vi "Initialize Front Panel.vi"(8 "error in (no error)":errorcluster, 11 "Subroutine Loop Dialog in":refnum<class "Subroutine Dialog.lvclass">) -> (0 "error out":errorcluster, 3 "For Loop Dialog out":refnum<class "Subroutine Dialog.lvclass">)   [LabVIEW 2019, in "Subroutine Dialog.lvclass"]
doc: "<License>\nCopyright © 2017 Composed Systems, LLC | All rights reserved\nwww.composed.io\n\nAuthor: Ethan Stern <ethan.stern@composed.io>\n\nThis software is provided \"AS IS\" WITHOUT WARRANTIES, either express or implied, AND IS FOR EDUCATIONAL PURPOSES ONLY.\n</License>"
uses:
  <vilib>/gpm_packages/@cs/Test-executive-builder/Source/Test Executive Builder Dialogs/Edit Subroutine Dialog/Subroutine Dialog.lvclass
  C:/Program Files/National Instruments/LabVIEW 2019/vi.lib/gpm_packages/@cs/popup-viewmanager/Source/Popup ViewManager/Popup ViewManager.lvclass
  <vilib>/gpm_packages/@cs/Test-executive-builder/Source/Test Executive Builder Dialogs/Edit Subroutine Dialog/Subroutine Dialog.lvclass/Subroutine Dialog.ctl
  <vilib>/gpm_packages/@cs/mva-viewable/Source/IViewable/IViewable Messages/Insert Front Panel Msg/Insert Front Panel Msg.lvclass/Insert Front Panel Msg.ctl
  <vilib>/ActorFramework/Message Enqueuer/Message Enqueuer.lvclass/Message Enqueuer.ctl
  <vilib>/gpm_packages/@cs/Test-executive-builder/Source/Test Executive Builder Dialogs/IAttribute Data Type View Messages/Set Value Msg/Set Value Msg.lvclass/Set Value Msg.ctl
  <vilib>/ActorFramework/Message Enqueuer/Enqueue.vi
  <vilib>/gpm_packages/@cs/mva-viewable/Source/IViewable/IViewable Messages/Insert Front Panel Msg/Insert Front Panel Msg.lvclass
  C:/Program Files/National Instruments/LabVIEW 2019/vi.lib/ActorFramework/Message/Message.lvclass
  <vilib>/gpm_packages/@cs/Test-executive-builder/Source/Test Executive Builder Dialogs/IAttribute Data Type View Messages/Set Value Msg/Set Value Msg.lvclass
  <vilib>/ActorFramework/Message Priority Queue/Priority Enqueue.vi
  <vilib>/gpm_packages/@cs/Test-executive-builder/Source/Test Executive Builder Dialogs/ITest Executive Builder Dialog/ITest Executive Builder Dialog.lvclass
  <vilib>/gpm_packages/@cs/popup-viewmanager/Source/Popup ViewManager/Popup ViewManager.lvclass
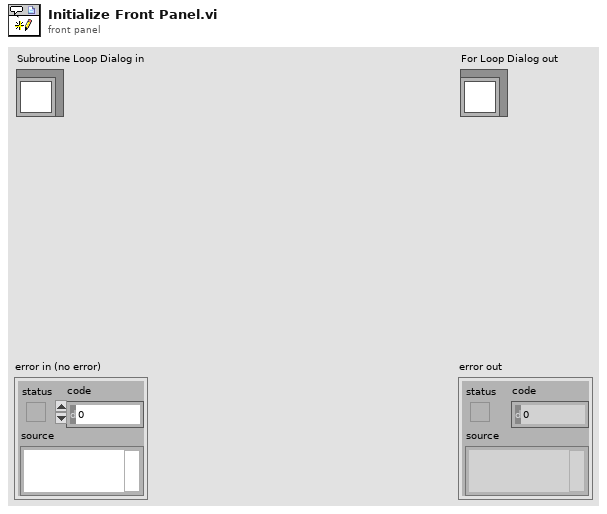
[diagram p1: front panel]
types:
  T1 = typedef "IViewable.lvlib/ProtectedSubpanel.lvclass/Protected Subpanel Reference.ctl" = refnum<data-value>
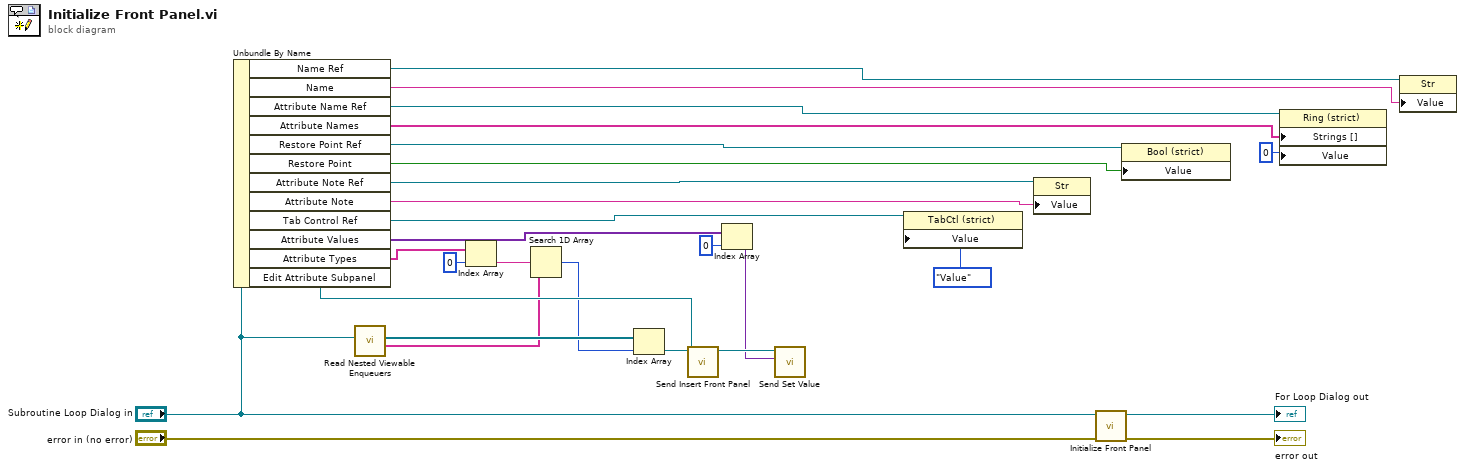
[diagram p0: block diagram]
diagram:
  n1 = Unbundle By Name("Subroutine Loop Dialog in") -> ("Name Ref"=w25:refnum<vi>, "Name"=w24:string, "Attribute Name Ref"=w22:refnum<vi>, "Attribute Names"=w21:string[], "Restore Point Ref"=w19:refnum<vi>, "Restore Point"=w18:bool, "Attribute Note Ref"=w17:refnum<vi>, "Attribute Note"=w16:string, "Tab Control Ref"=w11:refnum<vi>, "Attribute Values"=w2:variant[], "Attribute Types"=w9:string[], "Edit Attribute Subpanel"=w12:T1)
  n2 = call <vilib>:"Read Nested Viewable Enqueuers.vi"("Popup ViewManager in"="Subroutine Loop Dialog in") -> ("Viewable Names"=w7:string[], "Nested Enqueuers"=w14:refnum<class "Message Enqueuer.lvclass">[])  [unwired: 9 in]
  n3 = Index Array(array=w9, index=0) -> (element=w6:string)
  n4 = Search 1D Array(1D array=w7, element=w6) -> (index of element=w5:i32)  [unwired: 1 in]
  n5 = Index Array(array=w14, index=w5) -> (element=w13:refnum<class "Message Enqueuer.lvclass">)
  n6 = call <vilib>:"Send Insert Front Panel.vi"("Protected Subpanel"=w12, "Message Enqueuer"=w13) -> ("Message Enqueuer out"=w4:refnum<class "Message Enqueuer.lvclass">)  [unwired: 8 in, 1 out]
  n7 = Index Array(array=w2, index=0) -> (element=w1:variant)
  n8 = call <vilib>:"Send Set Value.vi"("Value"=w1, "Message Enqueuer"=w4) -> ()  [unwired: 8 in, 2 out]
  n9 = property class="TabCtl (strict)"(reference=w11, "Value"=enum32{"Value", "Pointer"}."Value") -> ()  [unwired: 1 in, 2 out]
  n10 = property class="Str"(reference=w17, "Value"=w16) -> ()  [unwired: 1 in, 2 out]
  n11 = call-parent "Initialize Front Panel.vi"("error in (no error)"="error in (no error)", "ITest Executive Builder Dialog in"="Subroutine Loop Dialog in") -> ("error out"=→"error out":errorcluster, "ITest Executive Builder Dialog out"=→"For Loop Dialog out":refnum<class "Subroutine Dialog.lvclass">)  [unwired: 8 in]
  n12 = property class="Bool (strict)"(reference=w19, "Value"=w18) -> ()  [unwired: 1 in, 2 out]
  n13 = property class="Ring (strict)"(reference=w22, "Strings []"=w21, "Value"=u16 0) -> ()  [unwired: 1 in, 2 out]
  n14 = property class="Str"(reference=w25, "Value"=w24) -> ()  [unwired: 1 in, 2 out]
